vi "Set Wavenumber.vi"(7 "Wave number":i32, 8 "error in (no error)":errorcluster, 11 "Comport":refnum<visa-resource-name>) -> (0 "error out":errorcluster, 2 "Set Success":bool, 3 "Comport 2":refnum<visa-resource-name>)   [LabVIEW 2018]
uses:
  <vilib>/Instr/_visa.llb/VISA Configure Serial Port (Instr).vi
panel:
  out "Numeric 2":i32
  out "Numeric":i32
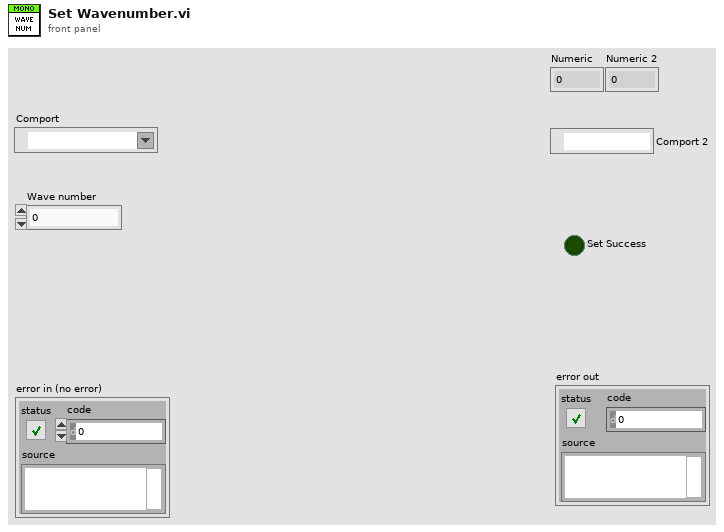
[diagram p1: front panel]
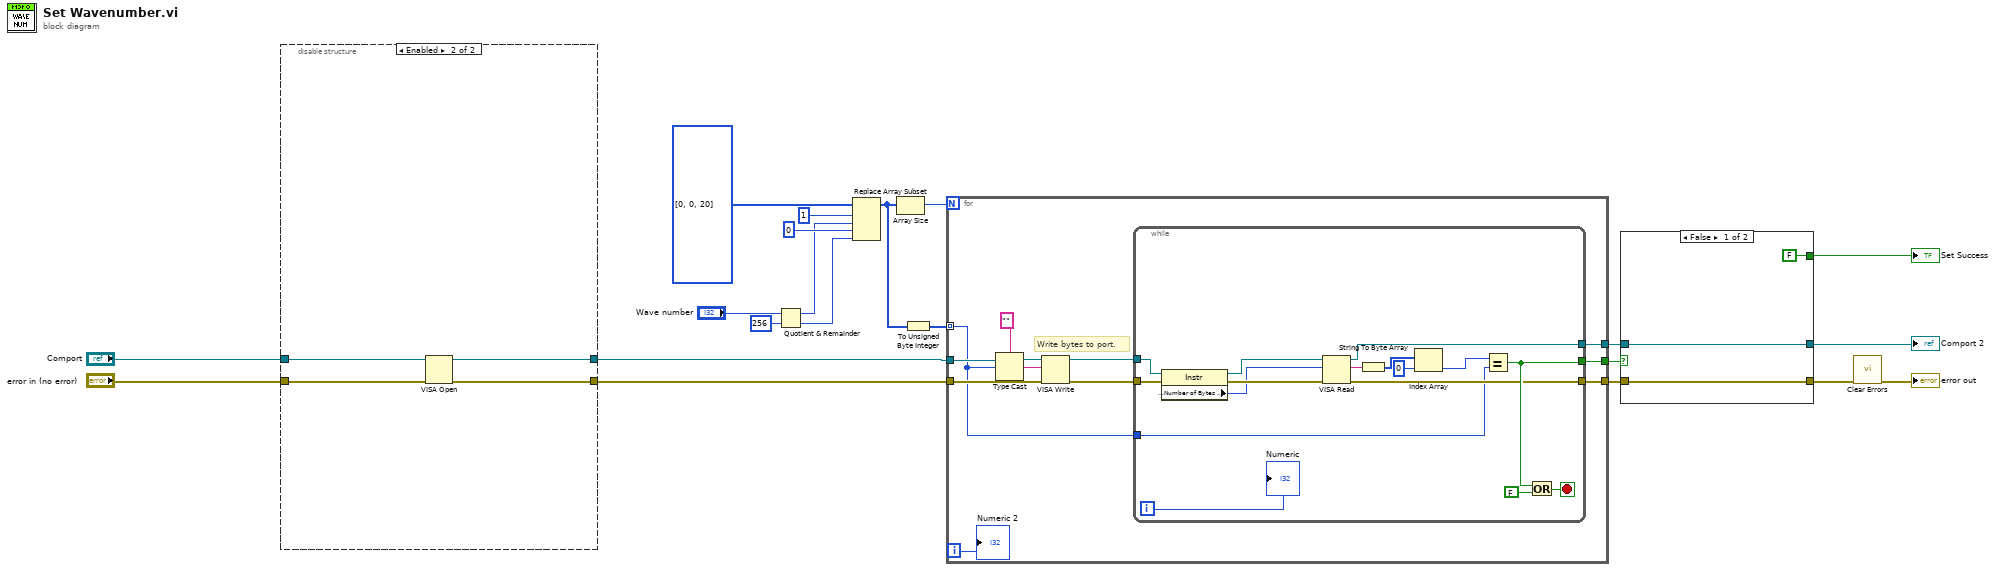
[diagram p0: block diagram]
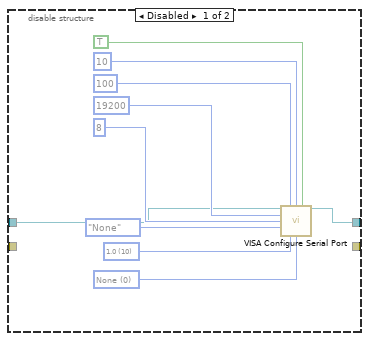
[diagram p2: hidden frame]
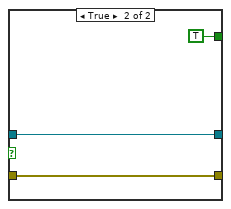
[diagram p3: hidden frame]
diagram:
  n1 = disable-structure shown="Enabled" {
    disable-tunnel: "Comport" -> [w23 w35]
    disable-tunnel: [w22 w34] -> w5
    disable-tunnel: "error in (no error)" -> [_ w33]
    disable-tunnel: [_ w32] -> w1
    frame Disabled {
      w31 = u16 0 items=["None", "XON/XOFF", "RTS/CTS", "XON/XOFF & RTS/CTS", "DTR/DSR", "XON/XOFF & DTR/DSR"] ("flow control (0:none)")
      w30 = u16 10 items=["1.0"=10, "1.5"=15, "2.0"=20] ("stop bits (10: 1 bit)")
      n2 = call-poly "VISA Configure Serial Port"("VISA resource name"=w23, "timeout (10sec)"=u32 100, "termination char\n(0xA = '\\n' = LF)"=u8 10 ("termination char\n(0xA = '\\n' = LF)"), "Enable Termination\nChar (T)"=TRUE ("Enable Termination\nChar (T)"), "baud rate (9600)"=u32 19200, "data bits (8)"=u16 8, "parity (0:none)"=enum16{"None", "Odd", "Even", "Mark", "Space"}."None", "stop bits (10: 1 bit)"=w30, "flow control (0:none)"=w31) -> ("VISA resource name out"=w22:refnum<visa-resource-name>)  [unwired: 5 in, 1 out]
    }
    frame Enabled {
      n3 = VISA Open(error in (no error)=w33, VISA resource name=w35) -> (VISA resource name=w34:refnum<visa-resource-name>, error out=w32:errorcluster)  [unwired: 3 in]
    }
  }
  n4 = Quotient & Remainder(x="Wave number", y=u32 256) -> (x-y*floor(x/y)=w3:u32, floor(x/y)=w4:u32)
  n5 = Replace Array Subset(array=i16[] [0, 0, 20], new element #1=w3, index #1=1 ("index"), new element #2=w4, index #2=0 ("index")) -> (w18:i16[])
  n6 = Array Size(array=w18) -> (size(s)=w12:i32)
  n7 = To Unsigned Byte Integer(number=w18) -> (unsigned 8bit integer=w7:u8[])
  n8 = for {
    N: w12 -> [_]
    tunnel: w7 -> [w37] mode=indexing
    tunnel: [w42] -> w13
    tunnel: [w41] -> w11
    tunnel: [w40] -> w10
    tunnel: w5 -> [w39]
    tunnel: w1 -> [w38]
    i -> [w36]
    # "Write bytes to port."
    n9 = Type Cast(type="", x=w37) -> (*(type *) &x=w45:string)
    n10 = VISA Write(VISA resource name=w39, write buffer=w45, error in (no error)=w38) -> (VISA resource name out=w44:refnum<visa-resource-name>, error out=w43:errorcluster)  [unwired: 1 out]
    n11 = while {
      tunnel: w44 -> [w55]
      tunnel: w43 -> [w54]
      tunnel: [w58] -> w42
      tunnel: [w57] -> w41
      tunnel: [w56] -> w40
      tunnel: w37 -> [w50]
      i -> [w47]
      stop <- w49 stop-if-true
      n12 = property class="Instr"(reference=w55, error in=w54) -> (reference out=w53:refnum<visa-resource-name>, error out=w52:errorcluster, "Serial Settings:Number of Bytes at Serial Port"=w51:u32)
      n13 = VISA Read(VISA resource name=w53, byte count=w51, error in (no error)=w52) -> (VISA resource name out=w57:refnum<visa-resource-name>, read buffer=w62:string, error out=w56:errorcluster)  [unwired: 1 out]
      n14 = String To Byte Array(string=w62) -> (unsigned byte array=w61:u8[])
      n15 = Index Array(array=w61, index=0) -> (element=w59:u8)
      n16 = Equal?(x=w59, y=w50) -> (x = y?=w58:bool)
      n17 = Or(x=w58, y=FALSE) -> (x .or. y?=w49:bool)
      "Numeric" <- w47
    }
    "Numeric 2" <- w36
  }
  n18 = case shown="False" w13 {
    tunnel: [FALSE TRUE] -> w14
    tunnel: w11 -> [w64 w67]
    tunnel: w10 -> [w63 w66]
    tunnel: [w64 w67] -> w21
    tunnel: [w63 w66] -> w20
    frame False {
    }
    frame True {
    }
  }
  "Comport 2" <- w21
  "Set Success" <- w14
  n19 = call <vilib>:"Clear Errors.vi"("error in (no error)"=w20) -> ("error out"=→"error out":errorcluster)  [unwired: 5 in, 1 out]
